vi "BCM-RF-GUI-3.2.vi"() -> ()   [LabVIEW 2020]
uses:
  <vilib>/Instr/_visa.llb/VISA Configure Serial Port (Instr).vi
panel:
  in  "BCM-RF-E COM Port":refnum<visa-resource-name>="COM3"
  out "Hold Delay BCM-RF":u32
  out "Scan Values":dbl[](array[numeric]) format="%.4f"
  out "Hold pre":u32=1
  out "Scan Delay":dbl[](array[numeric]) format="%.4f"
  in  "Graph Update Period [ms]":u32=100
  in  "Last Update Time":u32
  in  "Loop Update Period [ms]":i32=20
  out "Scan Read Delay Requested":bool
  out "Reconnect Str":string
  out "Retry Counter":i32
  out "COM Error":bool
  out "error out":errorcluster
  in  "error in":errorcluster
  out "BCM-RF-E Serial Number":i32
  out "Reset In Counter":bool
  out "Counter N RS232 In":u32
  in  "RS232 Out String":string
  out "N RS232 In":u32
  out "Comm Status":string
  in  "stop":bool
  in  "Window Tabs":T1(tab)
  in  "ADC On/Off":bool caption="On/Off"
  in  "Clear Chart":bool
  in  "ADC Average":u32(slide)=1 min=1 max=10000 step=1 scale=1.0..10000.0
  out "Trigger Received":bool
  in  "Save Configuration\nto BCM-RF-E":bool
  in  "Ucal":sgl=0.1234567 format="%_7g"
  in  "Qcal / Ical":sgl=0.1234567 format="%_7g"
  in  "Reverse\nTransfer Function":bool
  in  "Hold Delay":u32(slide) scale=0.0..255.0
  in  "CAL-FO Mode":bool caption="Enable\n \nDisable"
  in  "Measurement Mode":bool=TRUE caption="S&H\n\nT-C"
  in  "Trigger Mode":bool caption="On Board\n \nExternal"
  out "Data Graph":i32[](graph)
  out "String Iin":string="Iin = Ical * 10^(BCM Out / Ucal)"
  out "String Qin":string="Qin = Qcal * 10^(BCM Out / Ucal)"
  out "Scanning":bool
  out "TRG Count":u32
  in  "Trigger per Step":u32=1 min=1 max=100 step=1
  in  "Scan Step":u32=1 min=1 max=10 step=1
  in  "Scan Stop":u32=255 max=255 step=1
  in  "Scan Start":u32 max=255 step=1
  in  "Perform Scan":bool
  out "Scan Graph":cluster{dbl[], dbl[]}[](graph)
  out "Scan read delay":dbl
  in  "Available Measurement Modes":bool=TRUE caption="S&H / T-C\n \nT&H / T-C"
  in  "Internal Clock":bool=TRUE caption="Enable\n \nDisable"
  in  "Hold Delay Control":bool caption="Front Panel Trimmer\n \nDigital Hold Delay Line"
  in  "Trigger ADC Polarity":bool=TRUE caption="Positive Edge\n \nNegative Edge"
  in  "Re-Load BCM-RF-E Configuration":bool
  out "Data In":bool
  out "Data Out":bool
  out "Debit In":u32
  out "BCM-RF-E Identification String":string
  # "GUI v3.2"
  # "- Internal digital delay line"
  # "ns"
  # "ns"
  # "ns"
  # "The hold delay scan can be used to find the correct BCM-RF-E trigger timing, i.e. the timing of the signal apex.\nWhite dots show the raw data. After the scan a red line shows average values.\n\nAttention!\nThe scan is for information only. BCM-RF-E settings have to be manually set and saved in the main window."
  # "Switch positions according to Measurement Mode"
  # "Trigger\nMode"
  # "Hold Delay\nControl"
  # "Trigger\nReceived"
  # "Measurement\nMode"
  # "CAL-FO"
  # "On Board\nor \nExternal"
  # "Digital\nor\nFront Panel"
  # "Blinks on\nnew trigger"
  # "Disable"
  # "S&H"
  # "Disable"
  # "T-C"
  # "Not Used"
  # "Not Used"
  # "Not Used"
  # "Digital\nor\nFront Panel"
  # "Fixed to\nOn Board"
  # "Blinks on\nnew trigger"
  # "Enable"
  # "CAL-FO"
  # "Communication Status Details"
  # "On Board\nor \nExternal"
  # "Digital\nor\nFront Panel"
  # "Disable"
  # "Not Used"
  # "T&H"
  # "Special settings only required for special cases!"
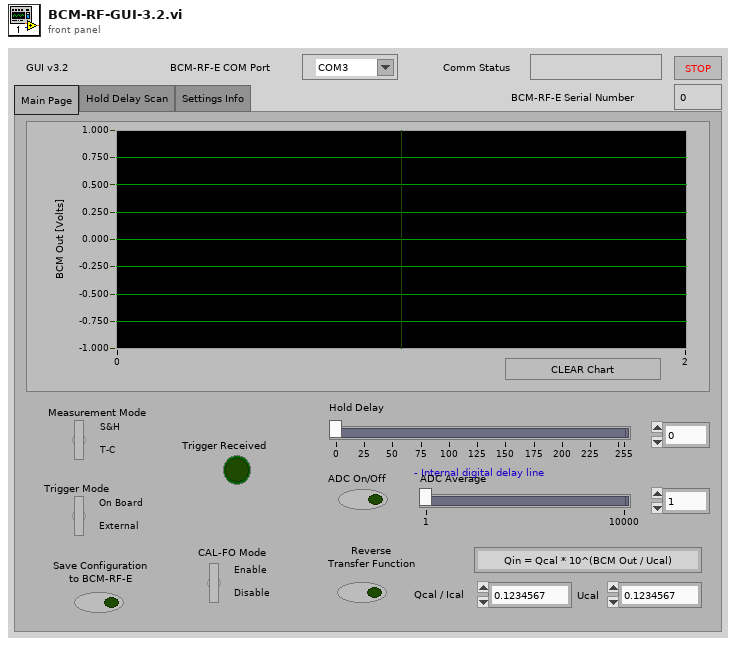
[diagram p1: front panel]
types:
  T1 = enum32{"Main Page", "Hold Delay Scan", "Settings Info"}
  T2 = enum8{"Enabled", "Disabled", "Disabled and Grayed Out"}
  T3 = cluster{"Scan Delay":dbl[], "Scan Values":dbl[]}[]
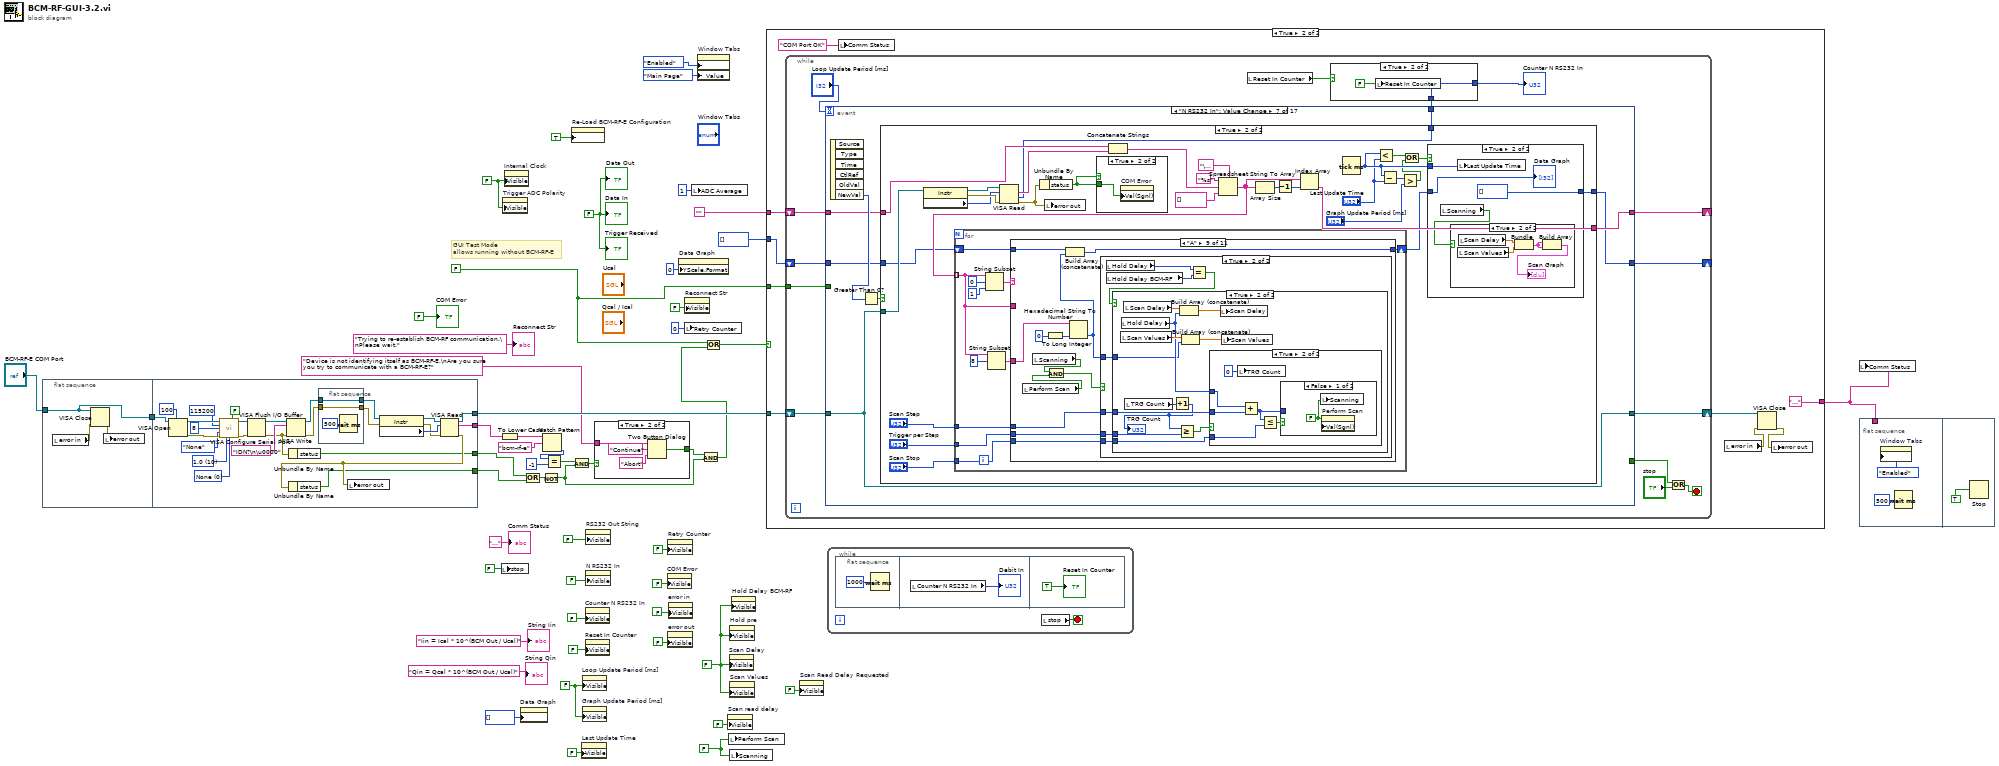
[diagram p0: block diagram]
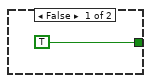
[diagram p2: hidden frame]
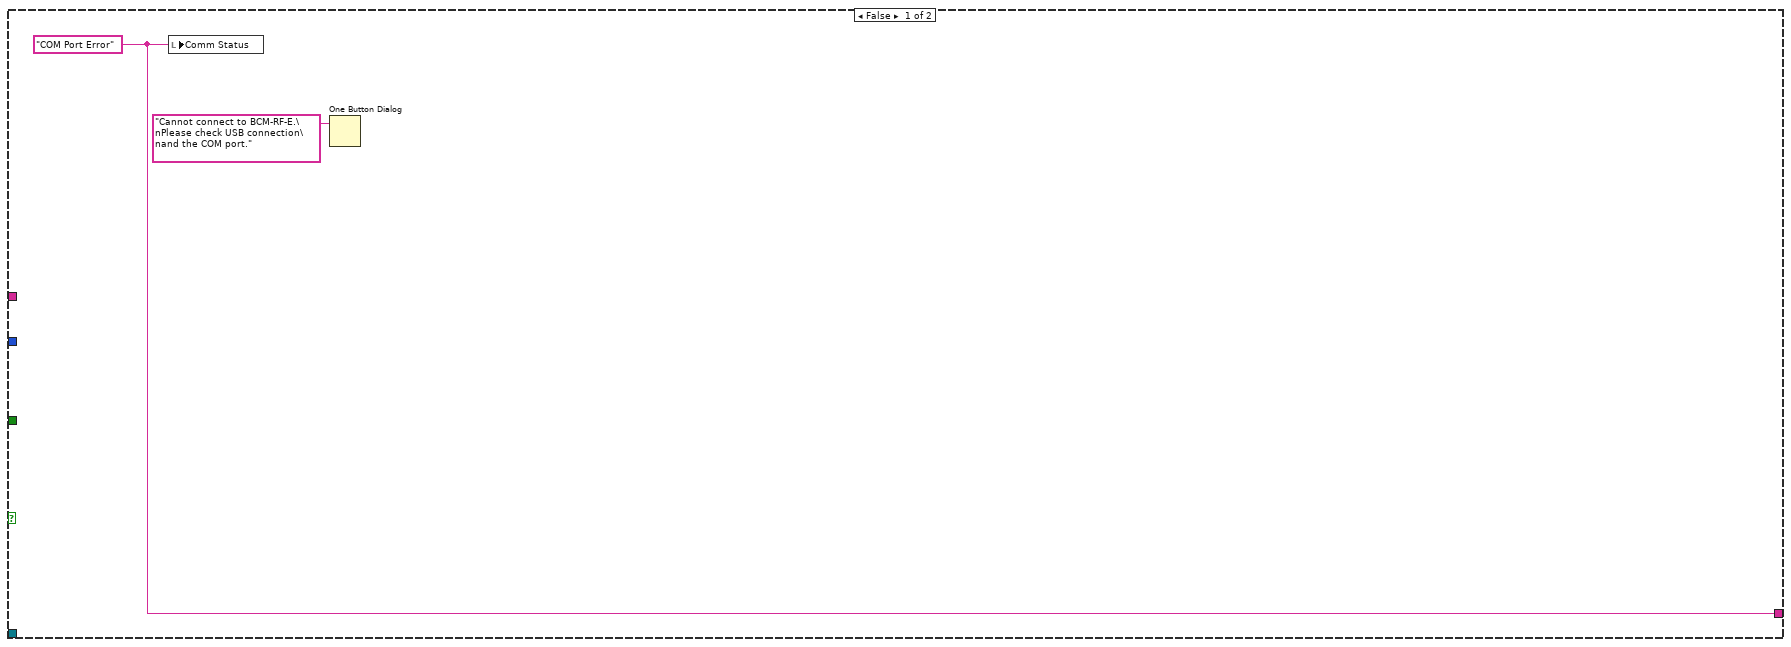
[diagram p3: hidden frame]
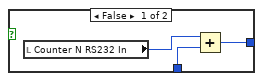
[diagram p4: hidden frame]
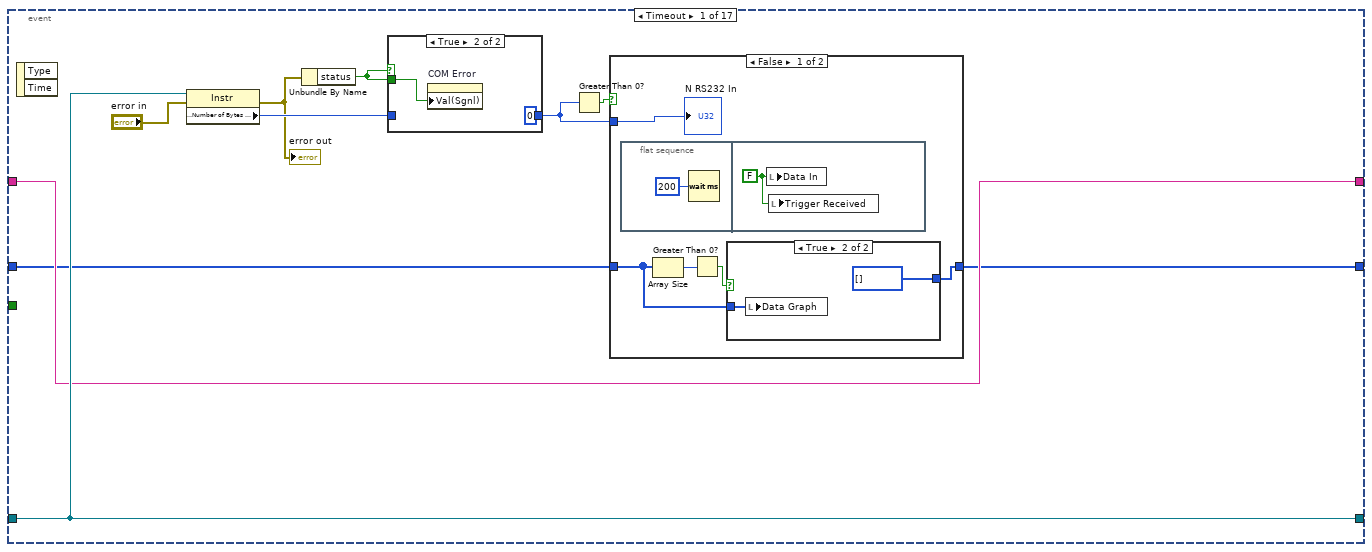
[diagram p5: hidden frame]
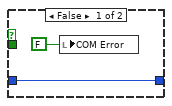
[diagram p6: hidden frame]
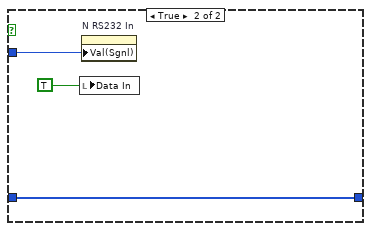
[diagram p8: hidden frame]
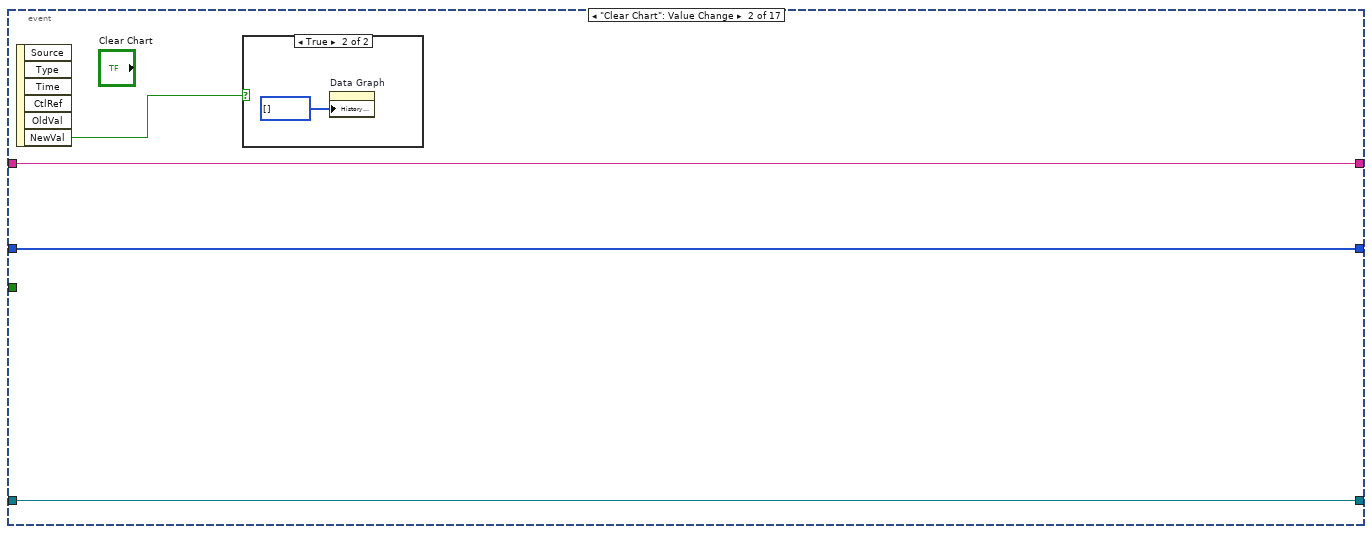
[diagram p9: hidden frame]
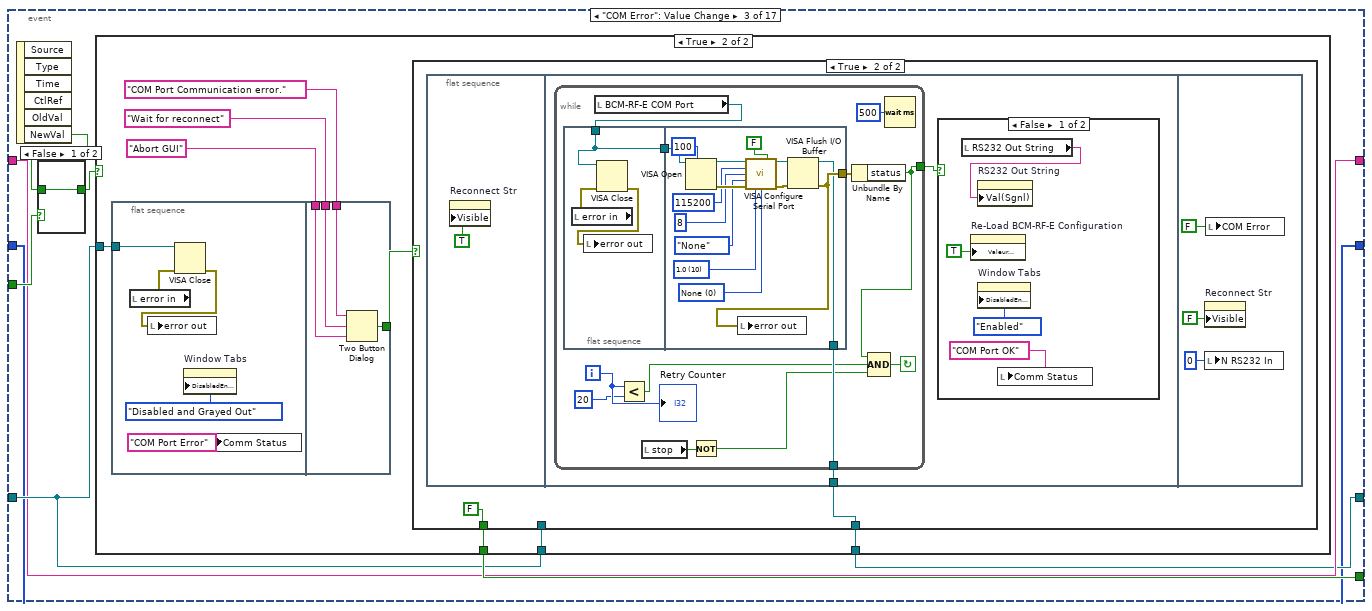
[diagram p11: hidden frame]
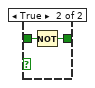
[diagram p12: hidden frame]
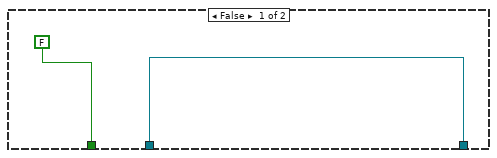
[diagram p13: hidden frame]
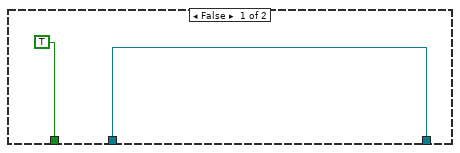
[diagram p14: hidden frame]
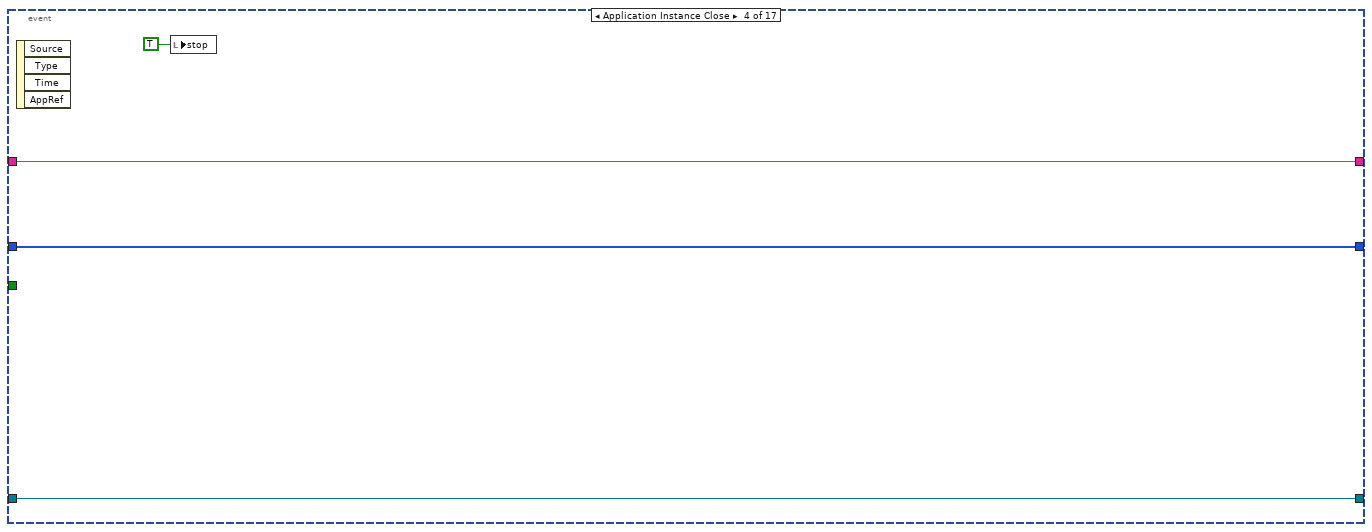
[diagram p16: hidden frame]
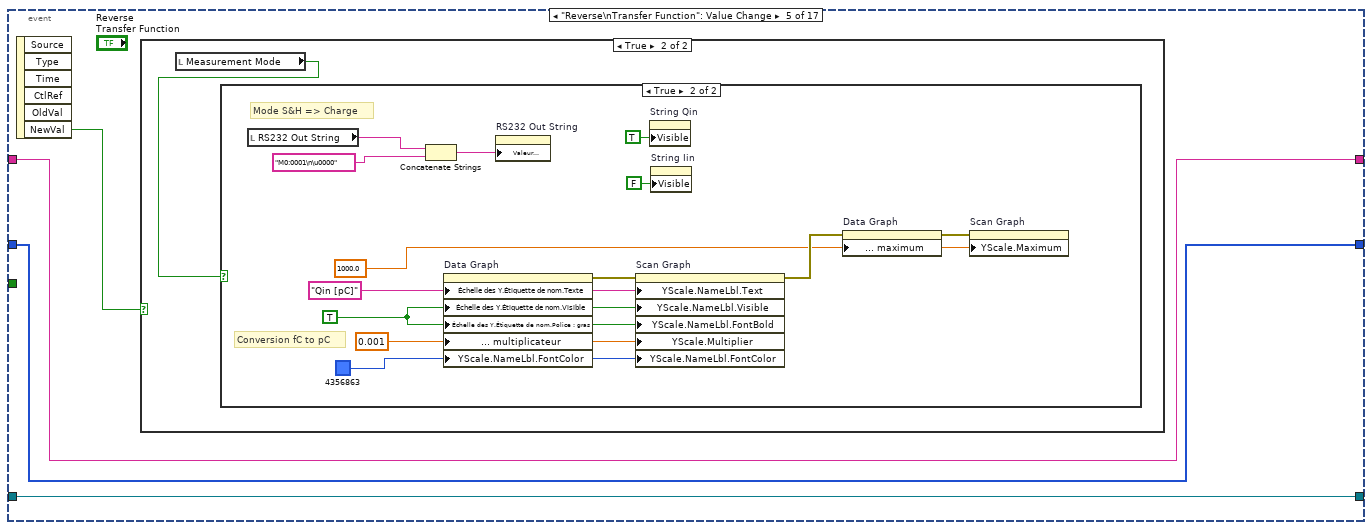
[diagram p17: hidden frame]
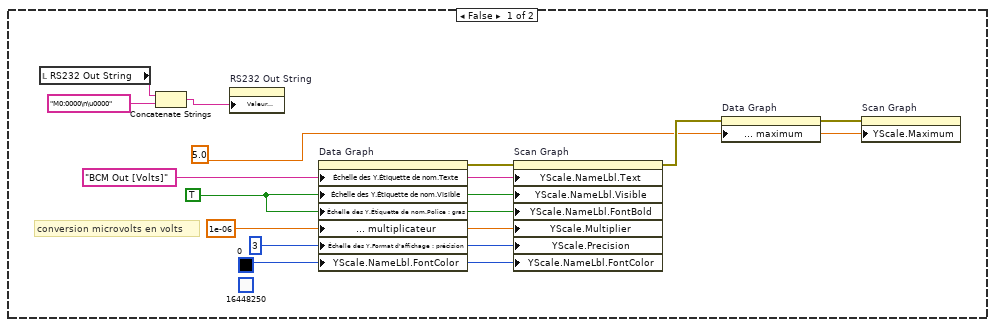
[diagram p18: hidden frame]
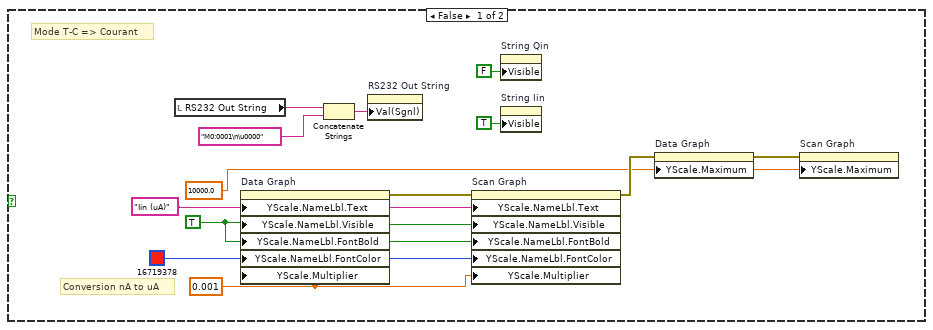
[diagram p19: hidden frame]
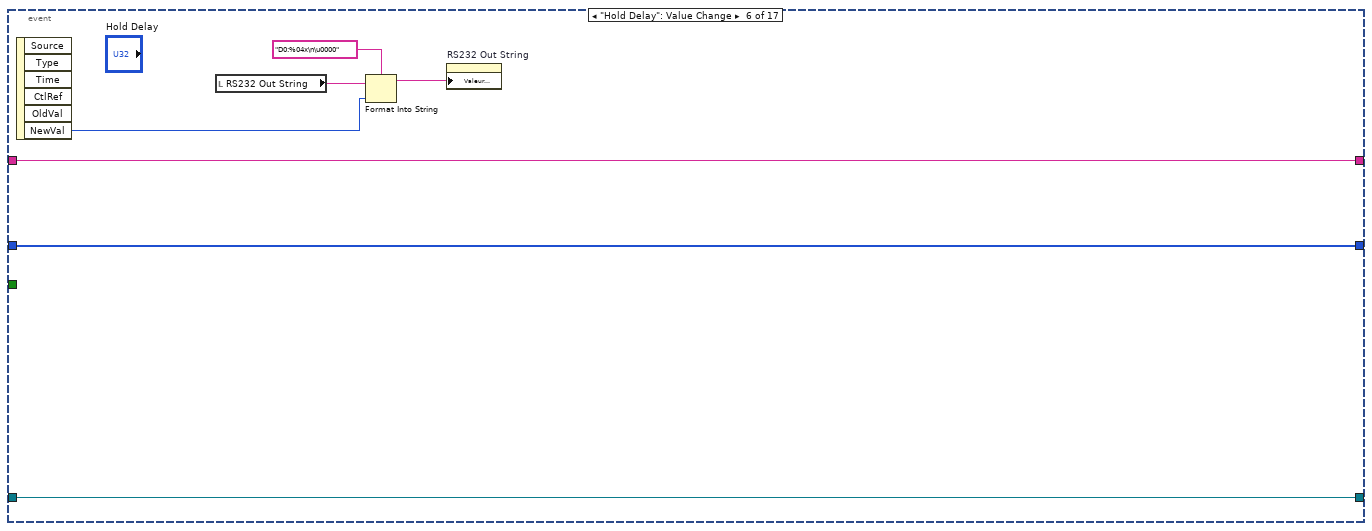
[diagram p20: hidden frame]
diagram:
  w19 = FALSE ("Visible")
  w13 = FALSE
  w22 = FALSE ("Visible")
  w42 = FALSE ("stop")
  w43 = FALSE ("stop")
  w26 = FALSE ("Data_In")
  # "GUI Test Mode\nallows running without BCM-RF-E"
  n1 = flat-sequence {
    tunnel: "BCM-RF-E COM Port" -> [w53]
    tunnel: [w53] -> w39
    tunnel: [w65] -> w9
    tunnel: [w68] -> w40
    tunnel: w39 -> [w81]
    tunnel: [w64] -> w10
    tunnel: [w63] -> w1
    frame #0 {
      n2 = local read "error in"() -> (w55:errorcluster)
      n3 = VISA Close(VISA resource name=w53, error in (no error)=w55) -> (error out=w54:errorcluster)
      n4 = local write "error out"(w54) -> ()
    }
    frame #1 {
      w72 = u16 0 items=["None", "XON/XOFF", "RTS/CTS", "XON/XOFF & RTS/CTS", "DTR/DSR", "XON/XOFF & DTR/DSR"] ("flow control (0:none)")
      w73 = u16 10 items=["1.0"=10, "1.5"=15, "2.0"=20] ("stop bits (10: 1 bit)")
      n5 = VISA Open(timeout (0)=u32 100 ("VISA Open timeout (0)"), VISA resource name=w81) -> (VISA resource name=w80:refnum<visa-resource-name>, error out=w77:errorcluster)  [unwired: 3 in]
      n6 = call-poly "VISA Configure Serial Port"("VISA resource name"=w80, "Enable Termination\nChar (T)"=FALSE ("Enable Termination\nChar (T)"), "baud rate (9600)"=u32 115200, "data bits (8)"=u16 8, "parity (0:none)"=enum16{"None", "Odd", "Even", "Mark", "Space"}."None", "error in (no error)"=w77, "stop bits (10: 1 bit)"=w73, "flow control (0:none)"=w72) -> ("VISA resource name out"=w79:refnum<visa-resource-name>, "error out"=w78:errorcluster)  [unwired: 6 out]
      n7 = VISA Flush I/O Buffer(VISA resource name=w79, error in (no error)=w78) -> (VISA resource name out=w70:refnum<visa-resource-name>, error out=w66:errorcluster)  [unwired: 1 in]
      n8 = VISA Write(VISA resource name=w70, write buffer="IDN?\n\u0000" ("Valeur (Signalisation)"), error in (no error)=w66) -> (VISA resource name out=w62:refnum<visa-resource-name>, error out=w61:errorcluster)  [unwired: 1 out]
      n9 = Unbundle By Name(w66) -> ("status"=w64:bool)
      n10 = flat-sequence {
        tunnel: w62 -> [w85]
        tunnel: [w85] -> w57
        tunnel: w61 -> [w84]
        tunnel: [w84] -> w56
        frame #0 {
          n11 = Wait (ms)(milliseconds to wait=u32 500) -> ()  [unwired: 1 out]
        }
      }
      n12 = property class="Instr"(reference=w57, error in=w56) -> (reference out=w60:refnum<visa-resource-name>, error out=w58:errorcluster, "Serial Settings:Number of Bytes at Serial Port"=w59:u32)
      n13 = VISA Read(VISA resource name=w60, byte count=w59, error in (no error)=w58) -> (VISA resource name out=w68:refnum<visa-resource-name>, read buffer=w63:string, error out=w67:errorcluster)  [unwired: 1 out]
      n14 = Unbundle By Name(w67) -> ("status"=w65:bool)
      n15 = local write "error out"(w67) -> ()
    }
  }
  n16 = To Lower Case(string=w1) -> (all lower case string=w16:string)
  n17 = local write "stop"(FALSE ("stop")) -> ()
  n18 = property on="Trigger ADC Polarity" class="Bool (strict)"("Visible"=w19) -> ()  [unwired: 2 in, 2 out]
  n19 = property on="Internal Clock" class="Bool (strict)"("Visible"=w19) -> ()  [unwired: 2 in, 2 out]
  n20 = property on="Data Graph" class="WFChart (strict)"("History Data"=i32[] []) -> ()  [unwired: 2 in, 2 out]
  n21 = Or(x=w10, y=w9) -> (x .or. y?=w8:bool)
  n22 = Not(x=w8) -> (.not. x?=w4:bool)
  n23 = Match Pattern(string=w16, regular expression="bcm-rf-e") -> (offset past match=w14:i32)  [unwired: 1 in, 3 out]
  n24 = Equal?(x=w14, y=-1) -> (x = y?=w7:bool)
  n25 = property on="Re-Load BCM-RF-E Configuration" class="Bool (strict)"("Valeur (Signalisation)"=TRUE ("Visible ?")) -> ()  [unwired: 2 in, 2 out]
  n26 = And(x=w7, y=w4) -> (x .and. y?=w6:bool)
  n27 = property on="Last Update Time" class="DigNum (strict)"("Visible"=FALSE) -> ()  [unwired: 2 in, 2 out]
  n28 = property on="Loop Update Period [ms]" class="DigNum (strict)"("Visible"=w22) -> ()  [unwired: 2 in, 2 out]
  n29 = property on="Graph Update Period [ms]" class="DigNum (strict)"("Visible"=w22) -> ()  [unwired: 2 in, 2 out]
  n30 = property on="Counter N RS232 In" class="DigNum (strict)"("Visible"=FALSE ("Visible ?")) -> ()  [unwired: 2 in, 2 out]
  n31 = property on="Reset In Counter" class="Bool (strict)"("Visible"=FALSE ("Visible ?")) -> ()  [unwired: 2 in, 2 out]
  n32 = property on="RS232 Out String" class="Str"("Visible"=FALSE ("Visible ?")) -> ()  [unwired: 2 in, 2 out]
  n33 = property on="N RS232 In" class="DigNum (strict)"("Visible"=FALSE ("Visible ?")) -> ()  [unwired: 2 in, 2 out]
  n34 = case shown="True" w6 {
    tunnel: "Device is not identifying itself as BCM-RF-E.\nAre you sure you try to communicate with a BCM-RF-E?" ("message") -> [_ w90]
    tunnel: [TRUE ("T button?") w87] -> w5
    frame False {
    }
    frame True {
      n35 = Two Button Dialog(message=w90, 1:"Abort" ("F button name (\"Cancel\")"), 2:"Continue" ("T button name (\"OK\")")) -> (T button?=w87:bool)
    }
  }
  n36 = property on="COM Error" class="Bool (strict)"("Visible"=FALSE ("Visible ?")) -> ()  [unwired: 2 in, 2 out]
  n37 = property on="Retry Counter" class="DigNum (strict)"("Visible"=FALSE ("Visible ?")) -> ()  [unwired: 2 in, 2 out]
  n38 = property on="error out" class="Clust (strict)"("Visible"=FALSE ("Visible ?")) -> ()  [unwired: 2 in, 2 out]
  n39 = property on="error in" class="Clust (strict)"("Visible"=FALSE ("Visible ?")) -> ()  [unwired: 2 in, 2 out]
  n40 = property on="Data Graph" class="WFChart (strict)"("YScale.Format"=u8 0 ("Y Scale.Display Format:Format")) -> ()  [unwired: 2 in, 2 out]
  n41 = local write "Retry Counter"(0 ("Retry Counter")) -> ()
  n42 = property on="Reconnect Str" class="Str"("Visible"=FALSE) -> ()  [unwired: 2 in, 2 out]
  n43 = local write "ADC Average"(u32 1 ("ADC Average")) -> ()
  n44 = property on="Window Tabs" class="TabCtl (strict)"("DisabledEnum"=T2."Enabled" ("Disabled"), "Value"=T1."Main Page" ("Window Tabs")) -> ()  [unwired: 2 in, 2 out]
  n45 = And(x=w5, y=w4) -> (x .and. y?=w3:bool)
  n46 = Or(x=w13, y=w3) -> (x .or. y?=w12:bool)
  n47 = property on="Scan read delay" class="DigNum (strict)"("Visible"=FALSE) -> ()  [unwired: 2 in, 2 out]
  n48 = local write "Perform Scan"(w42) -> ()
  n49 = property on="Scan Delay" class="Arr (strict)"("Visible"=w43) -> ()  [unwired: 2 in, 2 out]
  n50 = property on="Hold pre" class="DigNum (strict)"("Visible"=w43) -> ()  [unwired: 2 in, 2 out]
  n51 = property on="Scan Values" class="Arr (strict)"("Visible"=w43) -> ()  [unwired: 2 in, 2 out]
  n52 = local write "Scanning"(w42) -> ()
  n53 = property on="Hold Delay BCM-RF" class="DigNum (strict)"("Visible"=w43) -> ()  [unwired: 2 in, 2 out]
  n54 = case shown="True" w12 {
    tunnel: w40 -> [_ w97]
    tunnel: [w92 "..." ("Status")] -> w30
    tunnel: "" -> [_ w95]
    tunnel: i32[] [] -> [_ w93]
    tunnel: w13 -> [_ w94]
    frame False {
      w92 = "COM Port Error" ("Status")
      n55 = local write "Comm Status"(w92) -> ()
      n56 = One Button Dialog(message="Cannot connect to BCM-RF-E.\nPlease check USB connection\nand the COM port.") -> ()  [unwired: 1 in, 1 out]
    }
    frame True {
      n57 = while {
        shift-right: [w111] -> w96
        shift-left: w97 -> [w115]
        shift-right: [w105] -> _
        shift-left: w95 -> [w106]
        tunnel: w94 -> [w104]
        shift-right: [w102] -> _
        shift-left: w93 -> [w103]
        stop <- w114 stop-if-true
        n58 = event shown="[6] \"N RS232 In\": Value Change" {
          selector: _ -> [_ _ _ _ _ _ _ _ _ _ _ _ _ _ _ _ _]
          dyn-events: _ -> [_ _ _ _ _ _ _ _ _ _ _ _ _ _ _ _ _]
          timeout: "Loop Update Period [ms]" -> [_ _ _ _ _ _ _ _ _ _ _ _ _ _ _ _ _]
          tunnel: w115 -> [w125 w150 w159 w228 w232 w275 w281 w490 w498 w517 w525 w532 w609 w622 w637 w647 w702]
          tunnel: [_ _ w160 _ _ _ _ _ _ _ _ _ _ _ _ _ _] -> w112
          tunnel: [w125 w150 w154 w228 w232 w275 w281 w490 w498 w517 w525 w532 w609 w622 w637 w647 w702] -> w111
          tunnel: [_ _ _ _ _ _ w285 _ _ _ _ _ _ _ _ _ _] -> w107
          tunnel: w106 -> [w123 w149 w155 w227 w231 w274 w284 w489 w497 w513 w524 w533 w608 w621 w636 w646 w701]
          tunnel: [w123 w149 w155 w227 w231 w274 w283 w489 w497 w513 w524 w533 w608 w621 w636 w646 w701] -> w105
          tunnel: w103 -> [w122 w148 w153 w226 w230 w273 w282 w486 w496 w512 w523 w531 w607 w620 w633 w645 w700]
          tunnel: w104 -> [_ _ w156 _ _ _ _ _ _ _ _ _ _ _ _ _ _]
          tunnel: [w121 w148 w153 w226 w230 w273 w280 w486 w496 w512 w523 w531 w607 w620 w633 w645 w700] -> w102
          event Timeout {
            n59 = event-data() -> ()  [unwired: 3 out]
            n60 = property class="Instr"(reference=w125, error in="error in") -> (error out=w127:errorcluster, "Serial Settings:Number of Bytes at Serial Port"=w129:u32)  [unwired: 1 out]
            "error out" <- w127
            n61 = Unbundle By Name(w127) -> ("status"=w128:bool)
            n62 = case shown="True" w128 {
              tunnel: w128 -> [_ w134]
              tunnel: w129 -> [w132 _]
              tunnel: [w132 u32 0 ("Bytes at Port")] -> w126
              frame False {
                n63 = local write "COM Error"(FALSE ("COM Error")) -> ()
              }
              frame True {
                n64 = property on="COM Error" class="Bool (strict)"("Val(Sgnl)"=w134) -> ()  [unwired: 2 in, 2 out]
              }
            }
            n65 = Greater Than 0?(x=w126) -> (x > 0?=w130:bool)
            n66 = case shown="False" w130 {
              tunnel: w126 -> [w139 w147]
              tunnel: w122 -> [w137 w145]
              tunnel: [w135 w145] -> w121
              frame False {
                n67 = flat-sequence {
                  frame #0 {
                    n68 = Wait (ms)(milliseconds to wait=u32 200) -> ()  [unwired: 1 out]
                  }
                  frame #1 {
                    w144 = FALSE ("Data In")
                    n69 = local write "Data In"(w144) -> ()
                    n70 = local write "Trigger Received"(w144) -> ()
                  }
                }
                n71 = Array Size(array=w137) -> (size(s)=w138:i32)
                n72 = Greater Than 0?(x=w138) -> (x > 0?=w136:bool)
                n73 = case shown="True" w136 {
                  tunnel: w137 -> [w140 w142]
                  tunnel: [w140 i32[] []] -> w135
                  frame False {
                  }
                  frame True {
                    n74 = local write "Data Graph"(w142) -> ()
                  }
                }
                "N RS232 In" <- w139
              }
              frame True {
                n75 = local write "Data In"(TRUE ("Value (Signaling)")) -> ()
                n76 = property on="N RS232 In" class="DigNum (strict)"("Val(Sgnl)"=w147) -> ()  [unwired: 2 in, 2 out]
              }
            }
          }
          event "Clear Chart": Value Change {
            n77 = event-data() -> ("NewVal"=w151:bool)  [unwired: 6 out]
            n78 = case shown="True" w151 {
              frame False {
              }
              frame True {
                n79 = property on="Data Graph" class="WFChart (strict)"("History Data"=i32[] []) -> ()  [unwired: 2 in, 2 out]
              }
            }
          }
          event "COM Error": Value Change {
            n80 = event-data() -> ("NewVal"=w158:bool)  [unwired: 6 out]
            n81 = case shown="False" w156 {
              tunnel: w158 -> [w161 w163]
              tunnel: [w161 w162] -> w157
              frame False {
              }
              frame True {
                n82 = Not(x=w163) -> (.not. x?=w162:bool)
              }
            }
            n83 = case shown="True" w157 {
              tunnel: [FALSE ("stop") w173] -> w160
              tunnel: [w165 w172] -> w154
              tunnel: w159 -> [w165 w171]
              tunnel: w159 -> [_ w170]
              frame False {
              }
              frame True {
                n84 = flat-sequence {
                  tunnel: w170 -> [w176]
                  tunnel: [w182] -> w169
                  tunnel: "Abort GUI" ("F button name (\"Cancel\")") -> [w181]
                  tunnel: "Wait for reconnect" ("T button name (\"OK\")") -> [w180]
                  tunnel: "COM Port Communication error." ("message") -> [w179]
                  frame #0 {
                    n85 = local read "error in"() -> (w178:errorcluster)
                    n86 = VISA Close(VISA resource name=w176, error in (no error)=w178) -> (error out=w177:errorcluster)
                    n87 = local write "error out"(w177) -> ()
                    n88 = property on="Window Tabs" class="TabCtl (strict)"("DisabledEnum"=T2."Disabled and Grayed Out" ("Disabled")) -> ()  [unwired: 2 in, 2 out]
                    n89 = local write "Comm Status"("COM Port Error" ("Status")) -> ()
                  }
                  frame #1 {
                    n90 = Two Button Dialog(message=w179, 1:w181, 2:w180) -> (T button?=w182:bool)
                  }
                }
                n91 = case shown="True" w169 {
                  tunnel: [TRUE ("stop") FALSE] -> w173
                  tunnel: [w183 w185] -> w172
                  tunnel: w171 -> [w183 _]
                  frame False {
                  }
                  frame True {
                    n92 = flat-sequence {
                      tunnel: [w189] -> w185
                      frame #0 {
                        n93 = property on="Reconnect Str" class="Str"("Visible"=TRUE) -> ()  [unwired: 2 in, 2 out]
                      }
                      frame #1 {
                        n94 = while {
                          tunnel: [w202] -> w189
                          tunnel: [w195] -> w188
                          i -> [w204]
                          stop <- w197 continue-if-true
                          n95 = flat-sequence {
                            tunnel: w201 -> [w206]
                            tunnel: [w206] -> w200
                            tunnel: [w219] -> w203
                            tunnel: [w215] -> w202
                            tunnel: w200 -> [w216]
                            frame #0 {
                              n96 = local read "error in"() -> (w207:errorcluster)
                              n97 = VISA Close(VISA resource name=w206, error in (no error)=w207) -> (error out=w208:errorcluster)
                              n98 = local write "error out"(w208) -> ()
                            }
                            frame #1 {
                              w209 = u16 0 items=["None", "XON/XOFF", "RTS/CTS", "XON/XOFF & RTS/CTS", "DTR/DSR", "XON/XOFF & DTR/DSR"] ("flow control (0:none)")
                              w210 = u16 10 items=["1.0"=10, "1.5"=15, "2.0"=20] ("stop bits (10: 1 bit)")
                              n99 = VISA Open(timeout (0)=u32 100 ("VISA Open timeout (0)"), VISA resource name=w216) -> (VISA resource name=w217:refnum<visa-resource-name>, error out=w218:errorcluster)  [unwired: 3 in]
                              n100 = call-poly "VISA Configure Serial Port"("VISA resource name"=w217, "Enable Termination\nChar (T)"=FALSE ("Enable Termination\nChar (T)"), "baud rate (9600)"=u32 115200, "data bits (8)"=u16 8, "parity (0:none)"=enum16{"None", "Odd", "Even", "Mark", "Space"}."None", "error in (no error)"=w218, "stop bits (10: 1 bit)"=w210, "flow control (0:none)"=w209) -> ("VISA resource name out"=w222:refnum<visa-resource-name>, "error out"=w221:errorcluster)  [unwired: 6 out]
                              n101 = VISA Flush I/O Buffer(VISA resource name=w222, error in (no error)=w221) -> (VISA resource name out=w215:refnum<visa-resource-name>, error out=w219:errorcluster)  [unwired: 1 in]
                              n102 = local write "error out"(w219) -> ()
                            }
                          }
                          n103 = local read "BCM-RF-E COM Port"() -> (w201:refnum<visa-resource-name>)
                          n104 = Less?(x=w204, y=20) -> (x < y?=w194:bool)
                          n105 = local read "stop"() -> (w198:bool)
                          n106 = Not(x=w198) -> (.not. x?=w196:bool)
                          n107 = Unbundle By Name(w203) -> ("status"=w195:bool)
                          n108 = Compound Arithmetic op=AND(w195, w194, w196) -> (w197:bool)
                          n109 = Wait (ms)(milliseconds to wait=u32 500) -> ()  [unwired: 1 out]
                          "Retry Counter" <- w204
                        }
                        n110 = case shown="False" w188 {
                          frame False {
                            n111 = local read "RS232 Out String"() -> (w193:string)
                            n112 = property on="Re-Load BCM-RF-E Configuration" class="Bool (strict)"("Valeur (Signalisation)"=TRUE ("Value (Signaling)")) -> ()  [unwired: 2 in, 2 out]
                            n113 = property on="RS232 Out String" class="Str"("Val(Sgnl)"=w193) -> ()  [unwired: 2 in, 2 out]
                            n114 = property on="Window Tabs" class="TabCtl (strict)"("DisabledEnum"=T2."Enabled" ("Disabled")) -> ()  [unwired: 2 in, 2 out]
                            n115 = local write "Comm Status"("COM Port OK" ("Status")) -> ()
                          }
                          frame True {
                          }
                        }
                      }
                      frame #2 {
                        n116 = property on="Reconnect Str" class="Str"("Visible"=FALSE) -> ()  [unwired: 2 in, 2 out]
                        n117 = local write "N RS232 In"(u32 0 ("N Rs232 In")) -> ()
                        n118 = local write "COM Error"(FALSE ("COM Error")) -> ()
                      }
                    }
                  }
                }
              }
            }
          }
          event Application Instance Close {
            n119 = event-data() -> ()  [unwired: 5 out]
            n120 = local write "stop"(TRUE ("stop")) -> ()
          }
          event "Reverse\nTransfer Function": Value Change {
            n121 = event-data() -> ("NewVal"=w233:bool)  [unwired: 6 out]
            n122 = case shown="True" w233 {
              frame False {
                w238 = u32 0
                (unwired) u32 16448250
                w239 = u8 3 ("Échelle Y.Format & précision : précision")
                w240 = 1e-06 ("Échelle Y.Offset et multiplicateur : multiplicateur")
                w241 = TRUE ("Échelle Y.Étiquette de nom.Visible ?")
                w242 = "BCM Out [Volts]" ("Échelle Y.Étiquette de nom.Texte")
                w235 = 5.0 ("Échelle Y.Gamme : maximum")
                # "conversion microvolts en volts"
                n123 = local read "RS232 Out String"() -> (w245:string)
                n124 = Concatenate Strings(w245, "M0:0000\n\u0000" ("Valeur (Signalisation)")) -> (w243:string)
                n125 = property on="RS232 Out String" class="Str"("Valeur (Signalisation)"=w243) -> ()  [unwired: 2 in, 2 out]
                n126 = property on="Data Graph" class="WFChart (strict)"("Échelle des Y.Étiquette de nom.Texte"=w242, "Échelle des Y.Étiquette de nom.Visible"=w241, "Échelle des Y.Étiquette de nom.Police : gras"=w241, "Échelle des Y.Offset et multiplicateur : multiplicateur"=w240, "Échelle des Y.Format d'affichage : précision"=w239, "YScale.NameLbl.FontColor"=w238) -> (error out=w234:errorcluster)  [unwired: 2 in, 1 out]
                n127 = property on="Scan Graph" class="XYGraph (strict)"(error in=w234, "YScale.NameLbl.Text"=w242, "YScale.NameLbl.Visible"=w241, "YScale.NameLbl.FontBold"=w241, "YScale.Multiplier"=w240, "YScale.Precision"=w239, "YScale.NameLbl.FontColor"=w238) -> (error out=w237:errorcluster)  [unwired: 1 in, 1 out]
                n128 = property on="Data Graph" class="WFChart (strict)"(error in=w237, "Échelle des Y.Gamme : maximum"=w235) -> (error out=w236:errorcluster)  [unwired: 1 in, 1 out]
                n129 = property on="Scan Graph" class="XYGraph (strict)"(error in=w236, "YScale.Maximum"=w235) -> ()  [unwired: 1 in, 2 out]
              }
              frame True {
                n130 = local read "Measurement Mode"() -> (w246:bool)
                n131 = case shown="True" w246 {
                  frame False {
                    w251 = 0.001 ("Y Scale.Offset and Multiplier:Multiplier")
                    w253 = TRUE ("Y Scale.Name Label.Visible")
                    w254 = "Iin (uA)" ("Y Scale.Name Label.Text")
                    w247 = 10000.0 ("Y Scale.Range:Maximum")
                    w252 = u32 16719378
                    # "Conversion nA to uA"
                    # "Mode T-C => Courant"
                    n132 = local read "RS232 Out String"() -> (w256:string)
                    n133 = property on="Data Graph" class="WFChart (strict)"("YScale.NameLbl.Text"=w254, "YScale.NameLbl.Visible"=w253, "YScale.NameLbl.FontBold"=w253, "YScale.NameLbl.FontColor"=w252, "YScale.Multiplier"=w251) -> (error out=w249:errorcluster)  [unwired: 2 in, 1 out]
                    n134 = Concatenate Strings(w256, "M0:0001\n\u0000" ("Valeur (Signalisation)")) -> (w255:string)
                    n135 = property on="RS232 Out String" class="Str"("Val(Sgnl)"=w255) -> ()  [unwired: 2 in, 2 out]
                    n136 = property on="Scan Graph" class="XYGraph (strict)"(error in=w249, "YScale.NameLbl.Text"=w254, "YScale.NameLbl.Visible"=w253, "YScale.NameLbl.FontBold"=w253, "YScale.NameLbl.FontColor"=w252, "YScale.Multiplier"=w251) -> (error out=w248:errorcluster)  [unwired: 1 in, 1 out]
                    n137 = property on="String Qin" class="Str"("Visible"=FALSE) -> ()  [unwired: 2 in, 2 out]
                    n138 = property on="String Iin" class="Str"("Visible"=TRUE) -> ()  [unwired: 2 in, 2 out]
                    n139 = property on="Data Graph" class="WFChart (strict)"(error in=w248, "YScale.Maximum"=w247) -> (error out=w250:errorcluster)  [unwired: 1 in, 1 out]
                    n140 = property on="Scan Graph" class="XYGraph (strict)"(error in=w250, "YScale.Maximum"=w247) -> ()  [unwired: 1 in, 2 out]
                  }
                  frame True {
                    w264 = u32 4356863
                    w265 = 0.001 ("Échelle Y.Offset et multiplicateur : multiplicateur")
                    w266 = TRUE ("Échelle Y.Étiquette de nom.Visible ?")
                    w267 = "Qin [pC]" ("Échelle Y.Étiquette de nom.Texte")
                    w260 = 1000.0 ("Échelle Y.Gamme : maximum")
                    # "Mode S&H => Charge"
                    # "Conversion fC to pC"
                    n141 = local read "RS232 Out String"() -> (w272:string)
                    n142 = Concatenate Strings(w272, "M0:0001\n\u0000" ("Valeur (Signalisation)")) -> (w270:string)
                    n143 = property on="Data Graph" class="WFChart (strict)"("Échelle des Y.Étiquette de nom.Texte"=w267, "Échelle des Y.Étiquette de nom.Visible"=w266, "Échelle des Y.Étiquette de nom.Police : gras"=w266, "Échelle des Y.Offset et multiplicateur : multiplicateur"=w265, "YScale.NameLbl.FontColor"=w264) -> (error out=w263:errorcluster)  [unwired: 2 in, 1 out]
                    n144 = property on="RS232 Out String" class="Str"("Valeur (Signalisation)"=w270) -> ()  [unwired: 2 in, 2 out]
                    n145 = property on="Scan Graph" class="XYGraph (strict)"(error in=w263, "YScale.NameLbl.Text"=w267, "YScale.NameLbl.Visible"=w266, "YScale.NameLbl.FontBold"=w266, "YScale.Multiplier"=w265, "YScale.NameLbl.FontColor"=w264) -> (error out=w261:errorcluster)  [unwired: 1 in, 1 out]
                    n146 = property on="String Qin" class="Str"("Visible"=TRUE) -> ()  [unwired: 2 in, 2 out]
                    n147 = property on="String Iin" class="Str"("Visible"=FALSE) -> ()  [unwired: 2 in, 2 out]
                    n148 = property on="Data Graph" class="WFChart (strict)"(error in=w261, "Échelle des Y.Gamme : maximum"=w260) -> (error out=w262:errorcluster)  [unwired: 1 in, 1 out]
                    n149 = property on="Scan Graph" class="XYGraph (strict)"(error in=w262, "YScale.Maximum"=w260) -> ()  [unwired: 1 in, 2 out]
                  }
                }
              }
            }
          }
          event "Hold Delay": Value Change {
            n150 = event-data() -> ("NewVal"=w278:u32)  [unwired: 6 out]
            n151 = local read "RS232 Out String"() -> (w277:string)
            n152 = Format Into String(format string="D0:%04x\n\u0000" ("chaîne de format"), initial string=w277, w278) -> (resulting string=w276:string)  [unwired: 1 in, 1 out]
            n153 = property on="RS232 Out String" class="Str"("Valeur (Signalisation)"=w276) -> ()  [unwired: 2 in, 2 out]
          }
          event "N RS232 In": Value Change {
            n154 = event-data() -> ("NewVal"=w286:u32)  [unwired: 6 out]
            n155 = Greater Than 0?(x=w286) -> (x > 0?=w287:bool)
            n156 = case shown="True" w287 {
              tunnel: w281 -> [_ w311]
              tunnel: [u32 0 ("Bytes at Port") w305] -> w285
              tunnel: w284 -> [w289 w307]
              tunnel: [w289 w306] -> w283
              tunnel: [w288 w293] -> w280
              tunnel: w282 -> [w288 w292]
              frame False {
              }
              frame True {
                n157 = property class="Instr"(reference=w311) -> (reference out=w310:refnum<visa-resource-name>, error out=w309:errorcluster, "Serial Settings:Number of Bytes at Serial Port"=w308:u32)  [unwired: 1 in]
                n158 = VISA Read(VISA resource name=w310, byte count=w308, error in (no error)=w309) -> (read buffer=w320:string, return count=w305:u32, error out=w319:errorcluster)  [unwired: 1 out]
                n159 = Unbundle By Name(w319) -> ("status"=w318:bool)
                n160 = local write "error out"(w319) -> ()
                n161 = case shown="True" w318 {
                  tunnel: w318 -> [_ w330]
                  frame False {
                  }
                  frame True {
                    n162 = property on="COM Error" class="Bool (strict)"("Val(Sgnl)"=w330) -> ()  [unwired: 2 in, 2 out]
                  }
                }
                n163 = Concatenate Strings(w307, w320) -> (w317:string)
                n164 = Spreadsheet String To Array(delimiter (Tab)="\u0000", format string="%s", spreadsheet string=w317, array type (2D Dbl)=string[] []) -> (array=w301:string[])
                n165 = for {
                  tunnel: "Scan Step" -> [w341]
                  tunnel: "Scan Stop" -> [w340]
                  tunnel: "Trigger per Step" -> [w339]
                  tunnel: w301 -> [w334] mode=indexing
                  shift-right: [w331] -> w291
                  shift-left: w292 -> [w332]
                  n166 = String Subset(string=w334, offset (0)=0 ("index"), length (rest)=1 ("length")) -> (substring=w335:string)
                  n167 = String Subset(string=w334, offset (0)=8 ("index")) -> (substring=w333:string)  [unwired: 1 in]
                  n168 = case shown="\"A\"" w335 {
                    tunnel: w332 -> [w342 w347 w353 w360 w368 w382 w397 w425 w426 w479 w485]
                    tunnel: [w342 w347 w353 w360 w368 w382 w397 w425 w437 w479 w485] -> w331
                    tunnel: w341 -> [_ _ _ _ _ _ _ _ w436 _ _]
                    tunnel: w340 -> [_ _ _ _ _ _ _ _ w435 _ _]
                    tunnel: w339 -> [_ _ _ _ _ _ _ _ w434 _ _]
                    tunnel: w334 -> [_ _ _ _ w364 w378 w390 _ _ _ _]
                    tunnel: w333 -> [_ w346 w352 w359 w362 w376 w396 _ w433 w478 w484]
                    frame Default {
                    }
                    frame "T" {
                      n169 = Hexadecimal String To Number(string=w346) -> (number=w344:u32)  [unwired: 2 in, 1 out]
                      n170 = Equal To 0?(x=w344) -> (x = 0?=w345:bool)
                      n171 = case shown="True" w345 {
                        tunnel: w344 -> [w349 _]
                        tunnel: [TRUE ("ADC") FALSE ("ADC")] -> w343
                        frame False {
                          n172 = local write "ADC Average"(w349) -> ()
                        }
                        frame True {
                        }
                      }
                      n173 = local write "ADC On/Off"(w343) -> ()
                    }
                    frame "D" {
                      n174 = local read "Scanning"() -> (w355:bool)
                      n175 = Hexadecimal String To Number(string=w352) -> (number=w351:u32)  [unwired: 2 in, 1 out]
                      n176 = case shown="True" w355 {
                        tunnel: w351 -> [w356 w357]
                        frame False {
                          n177 = local write "Hold Delay"(w356) -> ()
                        }
                        frame True {
                          "Hold Delay BCM-RF" <- w357
                        }
                      }
                      "Scan Read Delay Requested" <- FALSE ("Scan Read Delay Requested")
                    }
                    frame "M" {
                      n178 = Hexadecimal String To Number(string=w359) -> (number=w358:u32)  [unwired: 2 in, 1 out]
                      n179 = Not Equal To 0?(x=w358) -> (x != 0?=w361:bool)
                      n180 = property on="Reverse\nTransfer Function" class="Bool (strict)"("Val(Sgnl)"=w361) -> ()  [unwired: 2 in, 2 out]
                    }
                    frame "V" {
                      n181 = Hexadecimal String To Number(string=w362) -> (number=w363:u32)  [unwired: 2 in, 1 out]
                      n182 = String Subset(string=w364, offset (0)=1 ("index"), length (rest)=1 ("length")) -> (substring=w365:string)
                      n183 = local read "Qcal / Ical"() -> (w375:sgl)
                      n184 = Decimal String To Number(string=w365) -> (number=w369:i32)  [unwired: 3 out]
                      n185 = Type Cast(type=u16[] [], x=w375) -> (*(type *) &x=w371:u16[])
                      n186 = Replace Array Subset(array=w371, new element=w363, index=w369) -> (w370:u16[])
                      n187 = Type Cast(type=sgl 0.0, x=w370) -> (*(type *) &x=w372:sgl)
                      n188 = local write "Qcal / Ical"(w372) -> ()
                    }
                    frame "W" {
                      n189 = Hexadecimal String To Number(string=w376) -> (number=w377:u32)  [unwired: 2 in, 1 out]
                      n190 = String Subset(string=w378, offset (0)=1 ("index"), length (rest)=1 ("length")) -> (substring=w379:string)
                      n191 = local read "Ucal"() -> (w389:sgl)
                      n192 = Decimal String To Number(string=w379) -> (number=w383:i32)  [unwired: 3 out]
                      n193 = Type Cast(type=u16[] [], x=w389) -> (*(type *) &x=w385:u16[])
                      n194 = Replace Array Subset(array=w385, new element=w377, index=w383) -> (w384:u16[])
                      n195 = Type Cast(type=sgl 0.0, x=w384) -> (*(type *) &x=w386:sgl)
                      n196 = local write "Ucal"(w386) -> ()
                    }
                    frame "I" {
                      n197 = String Subset(string=w390, offset (0)=0 ("index"), length (rest)=3 ("length")) -> (substring=w393:string)
                      n198 = Equal?(x=w393, y="IDN") -> (x = y?=w391:bool)
                      n199 = case shown="False" w391 {
                        tunnel: w396 -> [w403 _]
                        tunnel: w390 -> [_ w423]
                        frame False {
                          n200 = Hexadecimal String To Number(string=w403) -> (number=w404:u32)  [unwired: 2 in, 1 out]
                          n201 = And(x=w404, y=4) -> (x .and. y?=w408:u32)
                          n202 = And(x=w404, y=8) -> (x .and. y?=w411:u32)
                          n203 = And(x=w404, y=16) -> (x .and. y?=w410:u32)
                          n204 = And(x=w404, y=1) -> (x .and. y?=w412:u32)
                          n205 = And(x=w404, y=2) -> (x .and. y?=w409:u32)
                          n206 = Not Equal To 0?(x=w412) -> (x != 0?=w407:bool)
                          n207 = Not Equal To 0?(x=w409) -> (x != 0?=w399:bool)
                          n208 = Not Equal To 0?(x=w408) -> (x != 0?=w402:bool)
                          n209 = Not Equal To 0?(x=w411) -> (x != 0?=w406:bool)
                          n210 = Not Equal To 0?(x=w410) -> (x != 0?=w405:bool)
                          n211 = local write "Hold Delay Control"(w406) -> ()
                          n212 = local write "Trigger ADC Polarity"(w405) -> ()
                          n213 = local write "Trigger Mode"(w407) -> ()
                          n214 = case shown="False" w399 {
                            tunnel: w402 -> [w418 _]
                            tunnel: [w418 w420] -> w401
                            tunnel: [w419 w420] -> w400
                            tunnel: [w418 w420] -> w398
                            frame False {
                              n215 = Not(x=w418) -> (.not. x?=w419:bool)
                            }
                            frame True {
                              w420 = TRUE
                            }
                          }
                          n216 = local write "Measurement Mode"(w398) -> ()
                          n217 = local write "Internal Clock"(w401) -> ()
                          n218 = property on="Available Measurement Modes" class="Bool (strict)"("Val(Sgnl)"=w400) -> ()  [unwired: 2 in, 2 out]
                        }
                        frame True {
                          n219 = String Subset(string=w423, offset (0)=4) -> (substring=→"BCM-RF-E Identification String":string)  [unwired: 1 in]
                        }
                      }
                    }
                    frame "!" {
                      n220 = local write "Trigger Received"(TRUE ("Trigger Received")) -> ()
                    }
                    frame "A" {
                      n221 = local read "Perform Scan"() -> (w431:bool)
                      n222 = local read "Scanning"() -> (w430:bool)
                      n223 = To Long Integer(number=0 ("default (0 U32)")) -> (32bit integer=w427:i32)
                      n224 = And(x=w430, y=w431) -> (x .and. y?=w429:bool)
                      n225 = Hexadecimal String To Number(string=w433, default (0uL)=w427) -> (number=w432:i32)  [unwired: 1 in, 1 out]
                      n226 = Build Array (concatenate)(w426, w432) -> (w437:i32[])
                      n227 = case shown="True" w429 {
                        tunnel: w432 -> [_ w444]
                        tunnel: w436 -> [_ w440]
                        tunnel: w435 -> [_ w439]
                        tunnel: w434 -> [_ w438]
                        frame False {
                        }
                        frame True {
                          n228 = local read "Hold Delay"() -> (w441:u32)
                          n229 = local read "Hold Delay BCM-RF"() -> (w443:u32)
                          n230 = Equal?(x=w441, y=w443) -> (x = y?=w442:bool)
                          n231 = case shown="True" w442 {
                            tunnel: w444 -> [_ w463]
                            tunnel: w440 -> [_ w461]
                            tunnel: w439 -> [_ w460]
                            tunnel: w438 -> [_ w458]
                            frame False {
                              n232 = local read "Scan read delay"() -> (w449:dbl)
                              n233 = Greater Than 0?(x=w449) -> (x > 0?=w447:bool)
                              n234 = local read "Scan Read Delay Requested"() -> (w445:bool)
                              n235 = Not(x=w445) -> (.not. x?=w448:bool)
                              n236 = And(x=w447, y=w448) -> (x .and. y?=w446:bool)
                              n237 = case shown="True" w446 {
                                frame False {
                                }
                                frame True {
                                # "Hold Delay"
                                n238 = local read "Scan read delay"() -> (w452:dbl)
                                n239 = local read "RS232 Out String"() -> (w453:string)
                                n240 = Decrement(x=w452) -> (x-1=w451:dbl)
                                n241 = local write "Scan Read Delay Requested"(TRUE ("Scan Read Delay Requested")) -> ()
                                n242 = Concatenate Strings(w453, "D0?\n\u0000" ("Valeur (Signalisation)")) -> (w455:string)
                                n243 = local write "Scan read delay"(w451) -> ()
                                n244 = property on="RS232 Out String" class="Str"("Valeur (Signalisation)"=w455) -> ()  [unwired: 2 in, 2 out]
                                }
                              }
                            }
                            frame True {
                              n245 = local read "Scan Values"() -> (w466:dbl[])
                              n246 = local read "Hold Delay"() -> (w464:u32)
                              n247 = local read "Scan Delay"() -> (w467:dbl[])
                              n248 = local read "TRG Count"() -> (w462:u32)
                              n249 = Increment(x=w462) -> (x+1=w459:u32)
                              "TRG Count" <- w459
                              n250 = Greater Or Equal?(x=w459, y=w458) -> (x >= y?=w465:bool)
                              n251 = Build Array (concatenate)(w467, w464) -> (w456:dbl[])
                              n252 = Build Array (concatenate)(w466, w463) -> (w457:dbl[])
                              n253 = case shown="True" w465 {
                                tunnel: w464 -> [_ w470]
                                tunnel: w461 -> [_ w469]
                                tunnel: w460 -> [_ w468]
                                frame False {
                                }
                                frame True {
                                n254 = local write "TRG Count"(u32 0) -> ()
                                n255 = Add(x=w470, y=w469) -> (x+y=w472:u32)
                                n256 = Less Or Equal?(x=w472, y=w468) -> (x <= y?=w471:bool)
                                n257 = case shown="False" w471 {
                                tunnel: w472 -> [_ w476]
                                frame False {
                                w474 = FALSE
                                n258 = local write "Scanning"(w474) -> ()
                                n259 = property on="Perform Scan" class="Bool (strict)"("Val(Sgnl)"=w474) -> ()  [unwired: 2 in, 2 out]
                                }
                                frame True {
                                n260 = local write "Scan read delay"(10.0 ("Scan read delay")) -> ()
                                n261 = property on="Hold Delay" class="Slide (strict)"("Val(Sgnl)"=w476) -> ()  [unwired: 2 in, 2 out]
                                }
                                }
                                }
                              }
                              n262 = local write "Scan Delay"(w456) -> ()
                              n263 = local write "Scan Values"(w457) -> ()
                            }
                          }
                        }
                      }
                    }
                    frame "K" {
                      n264 = Hexadecimal String To Number(string=w478) -> (offset past number=w477:i32)  [unwired: 2 in, 1 out]
                      n265 = And(x=w477, y=1) -> (x .and. y?=w481:i32)
                      n266 = Not Equal To 0?(x=w481) -> (x != 0?=w480:bool)
                      n267 = property on="CAL-FO Mode" class="Bool (strict)"("Val(Sgnl)"=w480) -> ()  [unwired: 2 in, 2 out]
                    }
                    frame "S" {
                      n268 = Hexadecimal String To Number(string=w484) -> (number=→"BCM-RF-E Serial Number":u32)  [unwired: 2 in, 1 out]
                    }
                  }
                }
                n269 = Array Size(array=w301) -> (size(s)=w313:i32)
                n270 = Decrement(x=w313) -> (x-1=w312:i32)
                n271 = Index Array(array=w301, index=w312) -> (element=w306:string)
                n272 = Tick Count (ms)() -> (millisecond timer value=w298:u32)
                n273 = Less?(x=w298, y="Last Update Time") -> (x < y?=w296:bool)
                n274 = Subtract(x=w298, y="Last Update Time") -> (x-y=w300:u32)
                n275 = Greater?(x=w300, y="Graph Update Period [ms]") -> (0:w295:bool)
                n276 = Or(x=w296, y=w295) -> (x .or. y?=w294:bool)
                n277 = case shown="True" w294 {
                  tunnel: w298 -> [_ w325]
                  tunnel: w291 -> [w321 w322]
                  tunnel: [w321 i32[] []] -> w293
                  frame False {
                  }
                  frame True {
                    n278 = local read "Scanning"() -> (w324:bool)
                    n279 = case shown="True" w324 {
                      frame False {
                      }
                      frame True {
                        n280 = local read "Scan Values"() -> (w328:dbl[])
                        n281 = local read "Scan Delay"() -> (w327:dbl[])
                        n282 = Bundle("Scan Delay"=w327, "Scan Values"=w328) -> (w329:cluster{"Scan Delay":dbl[], "Scan Values":dbl[]})  [unwired: 1 in]
                        n283 = Build Array(w329, w329) -> (→"Scan Graph":T3)
                      }
                    }
                    n284 = local write "Last Update Time"(w325) -> ()
                    "Data Graph" <- w322
                  }
                }
              }
            }
          }
          event "ADC Average", "ADC On/Off": Value Change {
            n285 = event-data() -> ()  [unwired: 7 out]
            n286 = local read "RS232 Out String"() -> (w491:string)
            n287 = case shown="True" "ADC On/Off" {
              tunnel: [u32 0 ("ADC Average") "ADC Average"] -> w487
              frame False {
              }
              frame True {
              }
            }
            n288 = Format Into String(format string="T0:%04x\n\u0000" ("chaîne de format"), initial string=w491, w487) -> (resulting string=w492:string)  [unwired: 1 in, 1 out]
            n289 = property on="RS232 Out String" class="Str"("Valeur (Signalisation)"=w492) -> ()  [unwired: 2 in, 2 out]
          }
          event "Re-Load BCM-RF-E Configuration": Value Change {
            n290 = event-data() -> ("NewVal"=w500:bool)  [unwired: 6 out]
            n291 = case shown="True" w500 {
              frame False {
              }
              frame True {
                # "IDN String"
                # "Averaging"
                # "Cal Constants"
                # "Reverse Transfer"
                # "CAL-FO Mode"
                # "Hold Delay"
                # "Measurement Mode"
                # "Serial Number"
                n292 = local read "RS232 Out String"() -> (w502:string)
                n293 = Concatenate Strings(w502, "IDN?\n\u0000" ("Valeur (Signalisation)"), "S0?\n\u0000" ("Valeur (Signalisation)"), "I0?\n\u0000" ("Valeur (Signalisation)"), "D0?\n\u0000" ("Valeur (Signalisation)"), "M0?\n\u0000" ("Valeur (Signalisation)"), "K0?\n\u0000" ("Valeur (Signalisation)"), "V0?\n\u0000" ("Valeur (Signalisation)"), "W0?\n\u0000" ("Valeur (Signalisation)"), "T0?\n\u0000" ("Valeur (Signalisation)")) -> (w511:string)
                n294 = property on="RS232 Out String" class="Str"("Valeur (Signalisation)"=w511) -> ()  [unwired: 2 in, 2 out]
              }
            }
            n295 = local write "Re-Load BCM-RF-E Configuration"(FALSE ("Lecture\nEchantillonage")) -> ()
          }
          event "RS232 Out String": Value Change {
            n296 = event-data() -> ()  [unwired: 7 out]
            n297 = flat-sequence {
              frame #0 {
                n298 = local write "Data Out"(TRUE ("Data Out")) -> ()
              }
              frame #1 {
                n299 = Wait (ms)(milliseconds to wait=u32 50) -> ()  [unwired: 1 out]
              }
              frame #2 {
                n300 = local write "Data Out"(FALSE ("Data Out")) -> ()
              }
            }
            n301 = VISA Write(VISA resource name=w517, write buffer="RS232 Out String") -> (error out=w514:errorcluster)  [unwired: 1 in, 2 out]
            n302 = Unbundle By Name(w514) -> ("status"=w515:bool)
            n303 = local write "error out"(w514) -> ()
            n304 = case shown="False" w515 {
              tunnel: w515 -> [_ w522]
              frame False {
                n305 = local write "RS232 Out String"("") -> ()
              }
              frame True {
                n306 = property on="COM Error" class="Bool (strict)"("Val(Sgnl)"=w522) -> ()  [unwired: 2 in, 2 out]
              }
            }
          }
          event "Save Configuration\nto BCM-RF-E": Value Change {
            n307 = event-data() -> ("NewVal"=w527:bool)  [unwired: 6 out]
            n308 = local write "Save Configuration\nto BCM-RF-E"(FALSE ("Sauvegarde\nConfiguration")) -> ()
            n309 = case shown="True" w527 {
              frame False {
              }
              frame True {
                n310 = local read "RS232 Out String"() -> (w530:string)
                n311 = Concatenate Strings(w530, "E0:0001\n\u0000" ("Valeur (Signalisation)")) -> (w528:string)
                n312 = property on="RS232 Out String" class="Str"("Valeur (Signalisation)"=w528) -> ()  [unwired: 2 in, 2 out]
              }
            }
          }
          event "Trigger Mode", "Measurement Mode", "Internal Clock", "Hold Delay Control", "Trigger ADC Polarity": Value Change {
            # "Change mode only\nif not in CAL-FO mode"
            n313 = event-data() -> ()  [unwired: 7 out]
            n314 = local read "CAL-FO Mode"() -> (w536:bool)
            n315 = Equal?(x=w536, y=FALSE) -> (x = y?=w534:bool)
            n316 = case shown="True" w534 {
              frame False {
              }
              frame True {
                n317 = local read "Trigger Mode"() -> (w558:bool)
                n318 = local read "Measurement Mode"() -> (w550:bool)
                n319 = case shown="True" w550 {
                  tunnel: [FALSE TRUE] -> w537
                  tunnel: [w567 w590] -> w546
                  tunnel: [w566 w589] -> w545
                  tunnel: [w565 w588] -> w544
                  tunnel: [w564 w587] -> w543
                  tunnel: [w563 w586] -> w542
                  tunnel: [w562 w585] -> w541
                  tunnel: [w561 w584] -> w540
                  tunnel: [FALSE w583] -> w539
                  frame False {
                    # "Measurement Mode"
                    # "T-C Mode"
                    # "Internal clock"
                    n320 = local read "Reverse\nTransfer Function"() -> (w570:bool)
                    n321 = case shown="True" w570 {
                      tunnel: [u32 0 u32 16719378] -> w562
                      tunnel: [5.0 ("Échelle Y.Gamme : maximum") 10000.0 ("Y Scale.Range:Maximum")] -> w561
                      tunnel: [u8 3 ("Échelle Y.Format & précision : précision") u8 3 ("Échelle Y.Format & précision : précision")] -> w563
                      tunnel: [1e-06 ("Échelle Y.Offset et multiplicateur : multiplicateur") 0.001 ("Y Scale.Offset and Multiplier:Multiplier")] -> w564
                      tunnel: [w572 w579] -> w566
                      tunnel: [w572 w579] -> w565
                      tunnel: ["BCM Out [Volts]" ("Échelle Y.Étiquette de nom.Texte") "Iin (uA)" ("Y Scale.Name Label.Text")] -> w567
                      frame False {
                        w572 = TRUE ("Échelle Y.Étiquette de nom.Visible ?")
                        # "convert microvolts to volts"
                      }
                      frame True {
                        w579 = TRUE ("Y Scale.Name Label.Visible")
                        # "convert nA to uA"
                      }
                    }
                    n322 = property on="String Qin" class="Str"("Visible"=FALSE) -> ()  [unwired: 2 in, 2 out]
                    n323 = property on="String Iin" class="Str"("Visible"=TRUE) -> ()  [unwired: 2 in, 2 out]
                  }
                  frame True {
                    # "S&H or T&H Mode"
                    # "Internal clock"
                    n324 = local read "Available Measurement Modes"() -> (w583:bool)
                    n325 = local read "Reverse\nTransfer Function"() -> (w593:bool)
                    n326 = case shown="False" w593 {
                      tunnel: ["BCM Out [Volts]" ("Échelle Y.Étiquette de nom.Texte") "Qin [pC]" ("Échelle Y.Étiquette de nom.Texte")] -> w590
                      tunnel: [w599 w605] -> w588
                      tunnel: [w599 w605] -> w589
                      tunnel: [1e-06 ("Échelle Y.Offset et multiplicateur : multiplicateur") 0.001 ("Échelle Y.Offset et multiplicateur : multiplicateur")] -> w587
                      tunnel: [u8 3 ("Échelle Y.Format & précision : précision") u8 3 ("Échelle Y.Format & précision : précision")] -> w586
                      tunnel: [u32 0 u32 4356863] -> w585
                      tunnel: [5.0 ("Échelle Y.Gamme : maximum") 1000.0 ("Échelle Y.Gamme : maximum")] -> w584
                      frame False {
                        w599 = TRUE ("Échelle Y.Étiquette de nom.Visible ?")
                        # "convert microvolts to volts"
                      }
                      frame True {
                        w605 = TRUE ("Échelle Y.Étiquette de nom.Visible ?")
                        # "convert fC to pC"
                      }
                    }
                    n327 = property on="String Iin" class="Str"("Visible"=FALSE) -> ()  [unwired: 2 in, 2 out]
                    n328 = property on="String Qin" class="Str"("Visible"=TRUE) -> ()  [unwired: 2 in, 2 out]
                  }
                }
                n329 = local read "Trigger ADC Polarity"() -> (w551:bool)
                n330 = local read "Hold Delay Control"() -> (w552:bool)
                n331 = property on="Data Graph" class="WFChart (strict)"("YScale.NameLbl.Text"=w546, "YScale.NameLbl.Visible"=w545, "YScale.NameLbl.FontBold"=w544, "YScale.Multiplier"=w543, "YScale.Precision"=w542, "YScale.NameLbl.FontColor"=w541) -> (error out=w549:errorcluster)  [unwired: 2 in, 1 out]
                n332 = Build Array(w558, w539, w537, w552, w551) -> (w557:bool[])
                n333 = local write "Internal Clock"(w537) -> ()
                n334 = local read "RS232 Out String"() -> (w554:string)
                n335 = local write "Trigger Received"(FALSE ("Trigger ADC Out")) -> ()
                n336 = Boolean Array To Number(Boolean array=w557) -> (number=w555:u32)
                n337 = Format Into String(format string="I0:%04x\n\u0000" ("chaîne de format"), initial string=w554, w555) -> (resulting string=w553:string)  [unwired: 1 in, 1 out]
                n338 = property on="Scan Graph" class="XYGraph (strict)"(error in=w549, "YScale.NameLbl.Text"=w546, "YScale.NameLbl.Visible"=w545, "YScale.NameLbl.FontBold"=w544, "YScale.Multiplier"=w543, "YScale.Precision"=w542, "YScale.NameLbl.FontColor"=w541) -> (error out=w547:errorcluster)  [unwired: 1 in, 1 out]
                n339 = property on="Data Graph" class="WFChart (strict)"(error in=w547, "YScale.Maximum"=w540) -> (error out=w548:errorcluster)  [unwired: 1 in, 1 out]
                n340 = property on="Scan Graph" class="XYGraph (strict)"(error in=w548, "YScale.Maximum"=w540) -> ()  [unwired: 1 in, 2 out]
                n341 = property on="RS232 Out String" class="Str"("Valeur (Signalisation)"=w553) -> ()  [unwired: 2 in, 2 out]
              }
            }
          }
          event "Qcal / Ical": Value Change {
            n342 = event-data() -> ("NewVal"=w617:sgl)  [unwired: 6 out]
            n343 = local read "RS232 Out String"() -> (w619:string)
            n344 = Type Cast(type=u32 0, x=w617) -> (*(type *) &x=w615:u32)
            n345 = Split Number(x=w615) -> (hi(x)=w614:u16, lo(x)=w612:u16)
            n346 = Format Into String(format string="V1:%04x\n\u0000" ("chaîne de format"), initial string=w619, w614) -> (resulting string=w611:string)  [unwired: 1 in, 1 out]
            n347 = Format Into String(format string="V0:%04x\n\u0000" ("chaîne de format"), initial string=w611, w612) -> (resulting string=w610:string)  [unwired: 1 in, 1 out]
            n348 = property on="RS232 Out String" class="Str"("Valeur (Signalisation)"=w610) -> ()  [unwired: 2 in, 2 out]
          }
          event "Ucal": Value Change {
            n349 = event-data() -> ("NewVal"=w630:sgl)  [unwired: 6 out]
            n350 = local read "RS232 Out String"() -> (w632:string)
            n351 = Type Cast(type=u32 0, x=w630) -> (*(type *) &x=w628:u32)
            n352 = Split Number(x=w628) -> (hi(x)=w627:u16, lo(x)=w625:u16)
            n353 = Format Into String(format string="W1:%04x\n\u0000" ("chaîne de format"), initial string=w632, w627) -> (resulting string=w624:string)  [unwired: 1 in, 1 out]
            n354 = Format Into String(format string="W0:%04x\n\u0000" ("chaîne de format"), initial string=w624, w625) -> (resulting string=w623:string)  [unwired: 1 in, 1 out]
            n355 = property on="RS232 Out String" class="Str"("Valeur (Signalisation)"=w623) -> ()  [unwired: 2 in, 2 out]
          }
          event "CAL-FO Mode": Value Change {
            # "When changing CAL-FO mode, read also the BCM-RF state and hold delay"
            n356 = event-data() -> ("NewVal"=w642:bool)  [unwired: 6 out]
            n357 = case shown="True" w642 {
              tunnel: [T2."Enabled" ("Disabled") T2."Disabled and Grayed Out" ("Disabled")] -> w634
              frame False {
              }
              frame True {
              }
            }
            n358 = local read "RS232 Out String"() -> (w639:string)
            n359 = Boolean To (0,1)(Boolean="CAL-FO Mode") -> (0, 1=w641:i16)
            n360 = Format Into String(format string="K0:%04x\n\u0000I0?\n\u0000D0?\n\u0000" ("chaîne de format"), initial string=w639, w641) -> (resulting string=w638:string)  [unwired: 1 in, 1 out]
            n361 = property on="Measurement Mode" class="Bool (strict)"("DisabledEnum"=w634) -> ()  [unwired: 2 in, 2 out]
            n362 = property on="Trigger Mode" class="Bool (strict)"("DisabledEnum"=w634) -> ()  [unwired: 2 in, 2 out]
            n363 = property on="Available Measurement Modes" class="Bool (strict)"("DisabledEnum"=w634) -> ()  [unwired: 2 in, 2 out]
            n364 = property on="RS232 Out String" class="Str"("Valeur (Signalisation)"=w638) -> ()  [unwired: 2 in, 2 out]
          }
          event "Perform Scan": Value Change {
            n365 = event-data() -> ()  [unwired: 7 out]
            n366 = case shown="False" "Perform Scan" {
              frame False {
                w655 = 2
                n367 = local read "Scan Values"() -> (w658:dbl[])
                n368 = local read "Scan Delay"() -> (w657:dbl[])
                n369 = Initialize Array(0.0, 256, 2) -> (w662:dbl[][])
                n370 = for {
                  tunnel: w657 -> [w681] mode=indexing
                  tunnel: w658 -> [w682] mode=indexing
                  shift-right: [w677] -> w660
                  shift-left: w662 -> [w687]
                  n371 = Index Array(array=w687, index (row)=w681, index (col)=0) -> (element=w683:dbl)
                  n372 = Index Array(array=w687, index (row)=w681, index (col)=1) -> (element=w684:dbl)
                  n373 = Increment(x=w684) -> (x+1=w680:dbl)
                  n374 = Add(x=w682, y=w683) -> (x+y=w679:dbl)
                  n375 = Build Array(w679, w680) -> (w678:dbl[])
                  n376 = Replace Array Subset(array=w687, new element=w678, index (row)=w681) -> (w677:dbl[][])  [unwired: 1 in]
                }
                n377 = property on="Scan Graph" class="XYGraph (strict)"("XScale.ScaleFit"=w655, "YScale.ScaleFit"=w655, "Active Plot"=0, "Plot.Visible?"=TRUE, "Active Plot"=1, "Plot.Visible?"=TRUE) -> ()  [unwired: 2 in, 2 out]
                n378 = local read "Hold pre"() -> (w667:u32)
                n379 = local write "Scanning"(FALSE) -> ()
                n380 = for {
                  tunnel: w657 -> [w673] mode=indexing
                  tunnel: w660 -> [w674]
                  shift-right: [w668] -> w659
                  shift-left: dbl[] [] ("Scan Delay") -> [w670]
                  n381 = Index Array(array=w674, index (row)=w673, index (col)=0) -> (element=w672:dbl)
                  n382 = Index Array(array=w674, index (row)=w673, index (col)=1) -> (element=w671:dbl)
                  n383 = Divide(x=w672, y=w671) -> (x/y=w669:dbl)
                  n384 = Build Array (concatenate)(w670, w669) -> (w668:dbl[])
                }
                n385 = property on="Hold Delay" class="Slide (strict)"("Val(Sgnl)"=w667) -> ()  [unwired: 2 in, 2 out]
                n386 = Bundle("Scan Delay"=w657, "Scan Values"=w658) -> (w649:cluster{"Scan Delay":dbl[], "Scan Values":dbl[]})  [unwired: 1 in]
                n387 = Bundle("Scan Delay"=w657, "Scan Delay"=w659) -> (w650:cluster{"Scan Delay":dbl[], "Scan Delay":dbl[]})  [unwired: 1 in]
                n388 = Build Array(w650, w649) -> (w656:T3)
                n389 = local write "Scan Graph"(w656) -> ()
              }
              frame True {
                n390 = flat-sequence {
                  frame #0 {
                    w690 = 2
                    w689 = dbl[] [] ("Scan Delay")
                    n391 = local read "Hold Delay"() -> (→"Hold pre":u32)
                    n392 = local write "Hold Delay BCM-RF"(u32 123456) -> ()
                    n393 = local write "TRG Count"(0) -> ()
                    n394 = property on="Scan Graph" class="XYGraph (strict)"("XScale.ScaleFit"=w690, "YScale.ScaleFit"=w690, "Active Plot"=0, "Plot.Visible?"=FALSE, "Active Plot"=1, "Plot.Visible?"=TRUE) -> ()  [unwired: 2 in, 2 out]
                    "Scan Delay" <- w689
                    "Scan Values" <- w689
                    "Scan read delay" <- 10.0 ("Scan read delay")
                  }
                  frame #1 {
                    n395 = property on="Hold Delay" class="Slide (strict)"("Val(Sgnl)"="Scan Start") -> ()  [unwired: 2 in, 2 out]
                    "Scanning" <- TRUE
                  }
                }
              }
            }
          }
          event "Available Measurement Modes": Value Change {
            n396 = event-data() -> ()  [unwired: 7 out]
            n397 = local read "Measurement Mode"() -> (w703:bool)
            n398 = case shown="True" "Available Measurement Modes" {
              tunnel: ["T&H\n\nT-C" "S&H\n\nT-C"] -> w708
              frame False {
              }
              frame True {
              }
            }
            n399 = property on="Measurement Mode" class="Bool (strict)"("Val(Sgnl)"=w703) -> ()  [unwired: 2 in, 2 out]
            n400 = property on="Measurement Mode" class="Bool (strict)"("Caption.Text"=w708) -> (error out=w707:errorcluster)  [unwired: 2 in, 1 out]
            n401 = property on="Measurement Mode" class="Bool (strict)"(error in=w707, "Caption.Selection Start"=u32 3 ("Sous-titre.Sélection:Début"), "Caption.Selection End"=u32 5 ("Sous-titre.Sélection:Fin"), "Caption.FontSize"=u32 9 ("Sous-titre.Sélection:Fin")) -> ()  [unwired: 1 in, 2 out]
          }
        }
        n402 = local read "Reset In Counter"() -> (w109:bool)
        n403 = case shown="True" w109 {
          tunnel: w107 -> [w118 w119]
          tunnel: [w117 w119] -> w108
          frame False {
            n404 = local read "Counter N RS232 In"() -> (w116:u32)
            n405 = Add(x=w116, y=w118) -> (x+y=w117:u32)
          }
          frame True {
            n406 = local write "Reset In Counter"(FALSE ("Raz Cumul")) -> ()
          }
        }
        "Counter N RS232 In" <- w108
        n407 = Or(x=w112, y="stop") -> (x .or. y?=w114:bool)
      }
      n408 = local write "Comm Status"("COM Port OK" ("Status")) -> ()
      n409 = local read "error in"() -> (w99:errorcluster)
      n410 = VISA Close(VISA resource name=w96, error in (no error)=w99) -> (error out=w98:errorcluster)
      n411 = local write "error out"(w98) -> ()
    }
  }
  n412 = property on="Scan Read Delay Requested" class="Bool"("Visible"=FALSE) -> ()  [unwired: 2 in, 2 out]
  n413 = while {
    stop <- w712 stop-if-true
    n414 = flat-sequence {
      frame #0 {
        n415 = Wait (ms)(milliseconds to wait=u32 1000 ("attente (ms)")) -> ()  [unwired: 1 out]
      }
      frame #1 {
        n416 = local read "Counter N RS232 In"() -> (→"Debit In":u32)
      }
      frame #2 {
        "Reset In Counter" <- TRUE ("Raz Cumul")
      }
    }
    n417 = local read "stop"() -> (w712:bool)
  }
  n418 = local write "Comm Status"(w30) -> ()
  n419 = flat-sequence {
    tunnel: w30 -> [_]
    frame #0 {
      n420 = property on="Window Tabs" class="TabCtl (strict)"("DisabledEnum"=T2."Enabled" ("Disabled")) -> ()  [unwired: 2 in, 2 out]
      n421 = Wait (ms)(milliseconds to wait=u32 500) -> ()  [unwired: 1 out]
    }
    frame #1 {
      n422 = Stop(stop? (T)=TRUE ("stop ? (T)")) -> ()
    }
  }
  "Data In" <- w26
  "Data Out" <- w26
  "Comm Status" <- "..." ("Status")
  "Trigger Received" <- w26
  "String Iin" <- "Iin = Ical * 10^(BCM Out / Ucal)" ("String Iin")
  "String Qin" <- "Qin = Qcal * 10^(BCM Out / Ucal)" ("String Qin")
  "COM Error" <- FALSE ("COM Error")
  "Reconnect Str" <- "Trying to re-establish BCM-RF communication.\nPlease wait." ("Reconnect Str")
